vi "transcond_intensity_v2.vi"(10 "derivative bin size":dbl=20.0, 11 "Conductance":dbl[][](graph)) -> (3 "Transconductance":dbl[][](graph))   [LabVIEW 2016]
panel:
  in  "index":i32=1
  in  "dy/dx vs x":bool=TRUE
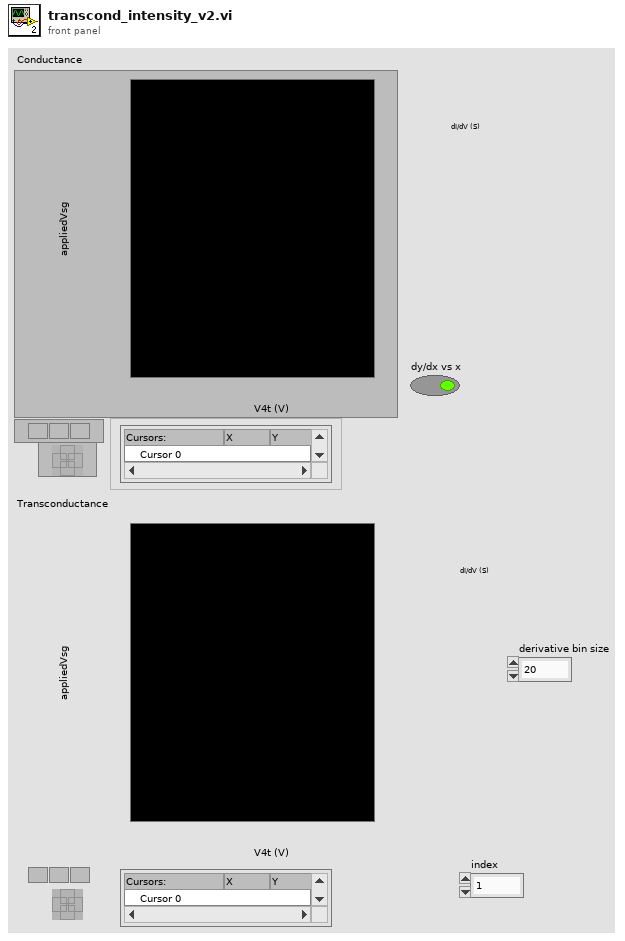
[diagram p1: front panel]
types:
  T1 = typedef "LVOffsetAndMultiplierTypeDef.ctl" = cluster{"Offset":dbl, "Multiplier":dbl}
  T2 = cluster{"Decimated Array":dbl[], "Decimated Array":dbl[]}
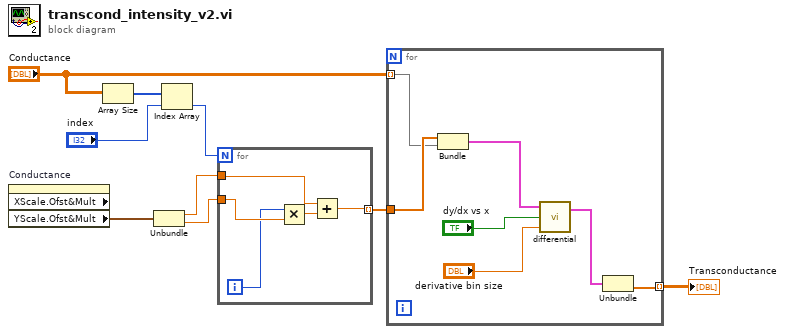
[diagram p0: block diagram]
diagram:
  n1 = property on="Conductance" class="IntGraph (strict)" props=["XScale", "Ofst&Mult", "YScale", "Ofst&Mult"]() -> ("YScale.Ofst&Mult"=w7:T1)  [unwired: 2 in, 3 out]
  n2 = Array Size(array="Conductance") -> (size(s)=w9:i32[])
  n3 = Unbundle(w7) -> ("Offset"=w6:dbl, "Multiplier"=w5:dbl)
  n4 = Index Array(array=w9, index="index") -> (element=w8:i32)
  n5 = for {
    N: w8 -> [_]
    tunnel: w6 -> [w12]
    tunnel: w5 -> [w14]
    tunnel: [w10] -> w4 mode=indexing
    i -> [w11]
    n6 = Multiply(x=w11, y=w14) -> (x*y=w13:dbl)
    n7 = Add(x=w12, y=w13) -> (x+y=w10:dbl)
  }
  n8 = for {
    tunnel: "Conductance" -> [w20] mode=indexing
    tunnel: w4 -> [w21]
    tunnel: [w15] -> w1 mode=indexing
    n9 = Bundle(w21, "Conductance"=w20) -> (w19:cluster{dbl[], "Conductance":dbl[]})  [unwired: 1 in]
    n10 = call <userlib>:"differential.vi"("Numeric"="derivative bin size", "dy/dx vs x"="dy/dx vs x", "A vs B 2"=w19) -> ("A vs B 3"=w16:T2)  [unwired: 1 in]
    n11 = Unbundle(w16) -> ("Decimated Array"=w15:dbl[])  [unwired: 1 out]
  }
  "Transconductance" <- w1
